vi "Get Aperture Time Info [DT].vi"(8 "error in (no error)":errorcluster, 11 "IVI_DMM in":refnum<class "IVI_DMM.lvclass">) -> (0 "error out":errorcluster, 1 "aperture time units":i32, 2 "aperture time (sec)":dbl format="%^.2e", 3 "IVI_DMM out":refnum<class "IVI_DMM.lvclass">)   [LabVIEW 2013, in "IVI_DMM.lvlib" / "IVI_DMM.lvclass"]
doc: "This VI returns additional information about the state of the instrument. Specifically, it returns the aperture time and the aperture time units.\n\nNote: \n\n(1) This VI is part of the IviDmmDeviceInfo [DI] extension group."
uses:
  IVI_DMM.lvclass
  IVI_DMM.lvclass/IVI_DMM.ctl
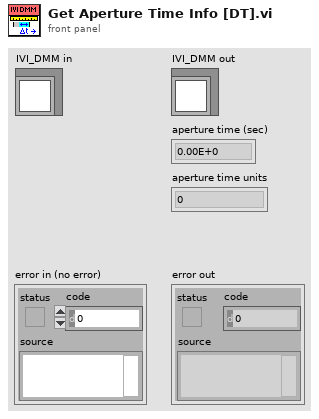
[diagram p1: front panel]
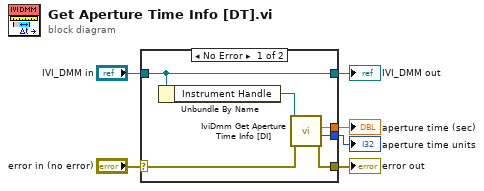
[diagram p0: block diagram]
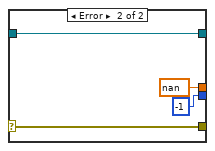
[diagram p2: hidden frame]
diagram:
  n1 = case shown="No Error" "error in (no error)" {
    selector: "error in (no error)" -> [w10 w16]
    tunnel: [w9 w16] -> w5
    tunnel: [w12 w15] -> w3
    tunnel: "IVI_DMM in" -> [w12 w15]
    tunnel: [w8 nan ("aperture time (sec)")] -> w2
    tunnel: [w7 -1 ("aperture time units")] -> w1
    frame No Error {
      n2 = Unbundle By Name(w12) -> ("Instrument Handle"=w11:refnum<k15>)
      n3 = call <vilib>:"IviDmm Get Aperture Time Info [DI].vi"("error in (no error)"=w10, "instrument handle"=w11) -> ("error out"=w9:errorcluster, "aperture time units"=w7:i32, "aperture time (sec)"=w8:dbl)  [unwired: 6 in, 1 out]
    }
    frame Error {
    }
  }
  "error out" <- w5
  "IVI_DMM out" <- w3
  "aperture time (sec)" <- w2
  "aperture time units" <- w1
